vi "ReadBatteryVoltage.vi"() -> (0 "Average Load Current":dbl, 1 "error wirte/read":errorcluster, 3 "Average Battery Voltage":dbl)   [LabVIEW 2021]
uses:
  <vilib>/DAQmx/write.llb/DAQmx Write (Digital U8 1Chan 1Samp).vi
  <vilib>/DAQmx/read.llb/DAQmx Read (Analog 2D DBL NChan NSamp).vi
  <vilib>/DAQmx/miscellaneous.llb/DAQmx Fill In Error Info.vi
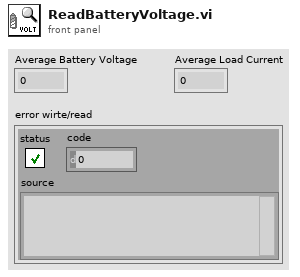
[diagram p1: front panel]
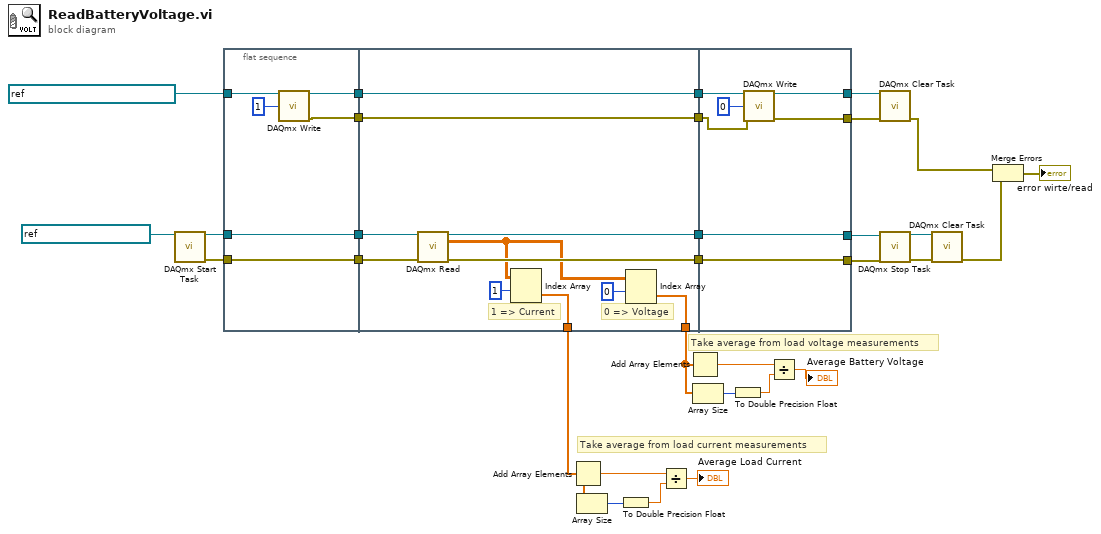
[diagram p0: block diagram]
diagram:
  # "Take average from load voltage measurements"
  # "Take average from load current measurements"
  n1 = call <vilib>:"DAQmx Start Task.vi"("task/channels in"=refnum<k21> "MeasurementsTask") -> ("task out"=w30:refnum<k21>, "error out"=w29:errorcluster)  [unwired: 13 in]
  n2 = flat-sequence {
    tunnel: w29 -> [w32]
    tunnel: w30 -> [w37]
    tunnel: [w37] -> w26
    tunnel: [w32] -> w25
    tunnel: refnum<k21> "ToggleLoadDigitalOutTask" ("task/channels in") -> [w35]
    tunnel: [w34] -> w21
    tunnel: [w33] -> w18
    tunnel: w26 -> [w46]
    tunnel: w25 -> [w45]
    tunnel: [w47] -> w24
    tunnel: [w48] -> w23
    tunnel: w21 -> [w44]
    tunnel: [w44] -> w20
    tunnel: [w43] -> w19
    tunnel: w18 -> [w43]
    tunnel: [w41] -> w12
    tunnel: [w39] -> w5
    tunnel: [w54] -> w15
    tunnel: [w55] -> w14
    tunnel: w24 -> [w55]
    tunnel: w23 -> [w54]
    tunnel: w20 -> [w49]
    tunnel: w19 -> [w52]
    tunnel: [w50] -> w17
    tunnel: [w51] -> w16
    frame #0 {
      n3 = call-poly <vilib>:"DAQmx Write.vi"("task/channels in"=w35, "data"=u8 1) -> ("task out"=w33:refnum<k21>, "error out"=w34:errorcluster)  [unwired: 11 in, 1 out]
    }
    frame #1 {
      # "0 => Voltage"
      # "1 => Current"
      n4 = call-poly <vilib>:"DAQmx Read.vi"("task/channels in"=w46, "error in"=w45) -> ("task out"=w47:refnum<k21>, "data"=w40:dbl[][], "error out"=w48:errorcluster)  [unwired: 11 in]
      n5 = Index Array(array=w40, index (row)=1) -> (element=w39:dbl[])  [unwired: 1 in]
      n6 = Index Array(array=w40, index (row)=0) -> (element=w41:dbl[])  [unwired: 1 in]
    }
    frame #2 {
      n7 = call-poly <vilib>:"DAQmx Write.vi"("task/channels in"=w52, "data"=u8 0, "error in"=w49) -> ("task out"=w50:refnum<k21>, "error out"=w51:errorcluster)  [unwired: 10 in, 1 out]
    }
  }
  n8 = Add Array Elements(numeric array=w5) -> (sum=w6:dbl)
  n9 = Array Size(array=w5) -> (size(s)=w3:i32)
  n10 = To Double Precision Float(number=w3) -> (double precision float=w4:dbl)
  n11 = Divide(x=w6, y=w4) -> (x/y=→"Average Load Current":dbl)
  n12 = Add Array Elements(numeric array=w12) -> (sum=w13:dbl)
  n13 = Array Size(array=w12) -> (size(s)=w2:i32)
  n14 = To Double Precision Float(number=w2) -> (double precision float=w1:dbl)
  n15 = Divide(x=w13, y=w1) -> (x/y=→"Average Battery Voltage":dbl)
  n16 = call <vilib>:"DAQmx Clear Task.vi"("task in"=w17, "error in"=w16) -> ("error out"=w8:errorcluster)  [unwired: 13 in]
  n17 = call <vilib>:"DAQmx Stop Task.vi"("task/channels in"=w14, "error in"=w15) -> ("task out"=w28:refnum<k21>, "error out"=w27:errorcluster)  [unwired: 12 in]
  n18 = call <vilib>:"DAQmx Clear Task.vi"("task in"=w28, "error in"=w27) -> ("error out"=w9:errorcluster)  [unwired: 13 in]
  n19 = Merge Errors(w8, w9) -> (→"error wirte/read":errorcluster)
